vi "Get Named Range of Sheet (String).vi"(8 "error in":errorcluster, 9 "Sheet Name":string, 10 "Named Range Identifier":string, 11 "SpreadsheetDocument":refnum<k24>) -> (0 "error out":errorcluster, 2 "Cells":string[][](array[string]), 3 "SpreadsheetDocument out":refnum<k24>)   [LabVIEW 2021, in "Open Xml.lvlib"]
uses:
  Open Xml.lvlib
  D:/git/Open-Xml-LabVIEW/Source/DocumentFormat.OpenXml.dll
  DocumentFormat.OpenXml.dll
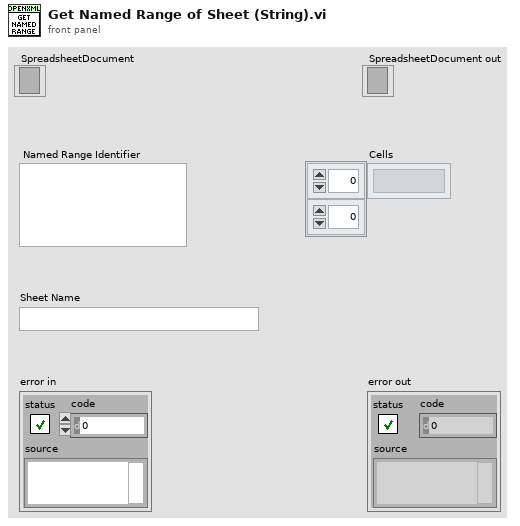
[diagram p1: front panel]
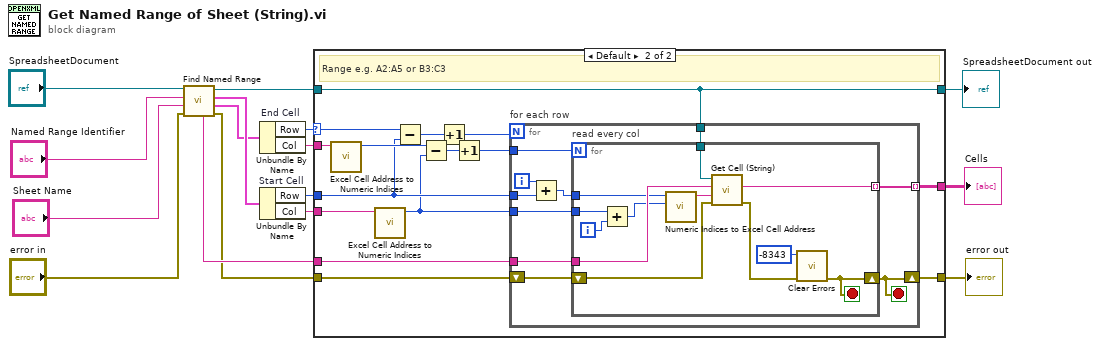
[diagram p0: block diagram]
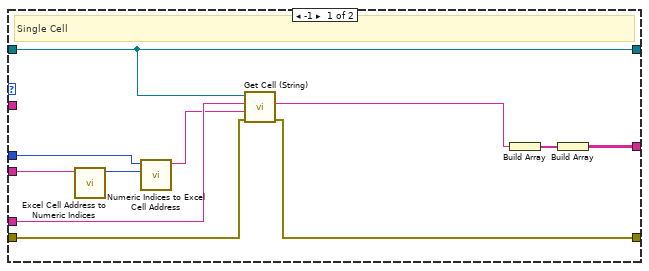
[diagram p2: hidden frame]
diagram:
  n1 = call "Find Named Range.vi"("error in"="error in", "Sheet Name"="Sheet Name", "Range Identifier"="Named Range Identifier", "SpreadsheetDocument"="SpreadsheetDocument") -> ("error out"=w6:errorcluster, "End Cell"=w14:cluster{"Col":string, "Row":i32}, "Start Cell"=w15:cluster{"Col":string, "Row":i32}, "SpreadsheetDocument"=w3:refnum<k24>, "Sheet Name"=w8:string)  [unwired: 3 in]
  n2 = Unbundle By Name "End Cell"(w14) -> ("Row"=w10:i32, "Col"=w12:string)
  n3 = Unbundle By Name "Start Cell"(w15) -> ("Row"=w9:i32, "Col"=w13:string)
  n4 = case shown="Default" w10 {
    selector: w10 -> [_ w37]
    tunnel: w13 -> [w26 w42]
    tunnel: w12 -> [_ w41]
    tunnel: w9 -> [w17 w34]
    tunnel: w8 -> [w27 w32]
    tunnel: [w19 w31] -> w7
    tunnel: w6 -> [w23 w30]
    tunnel: [w22 w29] -> w5
    tunnel: w3 -> [w18 w28]
    tunnel: [w18 w28] -> w2
    frame -1 {
      # "Single Cell"
      n5 = call "Excel Cell Address to Numeric Indices.vi"("Cell Name"=w26) -> ("Column Number"=w25:i32)  [unwired: 9 in, 1 out]
      n6 = call "Numeric Indices to Excel Cell Address.vi"("Column"=w25, "Row"=w17) -> ("Cell Address"=w24:string)  [unwired: 9 in]
      n7 = call "Get Cell (String).vi"("error in"=w23, "Cell Address"=w24, "Sheet Name"=w27, "SpreadsheetDocument"=w18) -> ("error out"=w22:errorcluster, "Value String"=w21:string)  [unwired: 5 in, 1 out]
      n8 = Build Array(w21) -> (w20:string[])
      n9 = Build Array(w20) -> (w19:string[][])
    }
    frame Default {
      # "Range e.g. A2:A5 or B3:C3"
      n10 = call "Excel Cell Address to Numeric Indices.vi"("Cell Name"=w41) -> ("Column Number"=w40:i32)  [unwired: 9 in, 1 out]
      n11 = call "Excel Cell Address to Numeric Indices.vi"("Cell Name"=w42) -> ("Column Number"=w33:i32)  [unwired: 9 in, 1 out]
      n12 = Subtract(x=w37, y=w34) -> (x-y=w36:i32)
      n13 = Subtract(x=w40, y=w33) -> (x-y=w38:i32)
      n14 = Increment(x=w36) -> (x+1=w35:i32)
      n15 = Increment(x=w38) -> (x+1=w39:i32)
      n16 = for "for each row" {
        N: w35 -> [_]
        tunnel: w39 -> [w52]
        tunnel: w34 -> [w49]
        tunnel: w33 -> [w51]
        tunnel: w32 -> [w50]
        tunnel: [w48] -> w31 mode=indexing
        shift-right: [w44] -> w29
        shift-left: w30 -> [w45]
        tunnel: w28 -> [w43]
        i -> [w46]
        stop <- w44 stop-if-true
        n17 = Add(x=w46, y=w49) -> (x+y=w47:i32)
        n18 = for "read every col" {
          N: w52 -> [_]
          tunnel: w51 -> [w62]
          tunnel: w50 -> [w64]
          tunnel: w47 -> [w61]
          tunnel: [w60] -> w48 mode=indexing
          shift-right: [w55] -> w44
          shift-left: w45 -> [w57]
          tunnel: w43 -> [w53]
          i -> [w58]
          stop <- w55 stop-if-true
          n19 = Add(x=w62, y=w58) -> (x+y=w59:i32)
          n20 = call "Numeric Indices to Excel Cell Address.vi"("Column"=w59, "Row"=w61) -> ("Cell Address"=w63:string)  [unwired: 9 in]
          n21 = call "Get Cell (String).vi"("error in"=w57, "Cell Address"=w63, "Sheet Name"=w64, "SpreadsheetDocument"=w53) -> ("error out"=w56:errorcluster, "Value String"=w60:string)  [unwired: 5 in, 1 out]
          n22 = call <vilib>:"Clear Errors.vi"("error in (no error)"=w56, "specific error code to clear (0: all)"=-8343) -> ("error out"=w55:errorcluster)  [unwired: 4 in, 1 out]
        }
      }
    }
  }
  "error out" <- w5
  "Cells" <- w7
  "SpreadsheetDocument out" <- w2
